vi "Set Exclusions By Path.vi"(8 "error in (no error)":errorcluster, 10 "Path exclusions":T1={"Exclude files from vi.lib"=TRUE, "Exclude files from instr.lib"=TRUE, "Exclude files from user.lib"=TRUE}, 11 "SDIST in":refnum<class "NI_AB_API_DSDIST.lvclass">) -> (0 "error out":errorcluster, 3 "SDIST out":refnum<class "NI_AB_API_DSDIST.lvclass">)   [LabVIEW 2020, in "NI_AB_API_DSDIST.lvclass"]
uses:
  <vilib>/AppBuilder/AB_API/DSDIST/NI_AB_API_DSDIST.lvclass
  <vilib>/AppBuilder/AB_API/common/AB_API Path Exclusions.ctl
  <vilib>/AppBuilder/AB_API/SDIST/NI_AB_API_SDIST.lvclass
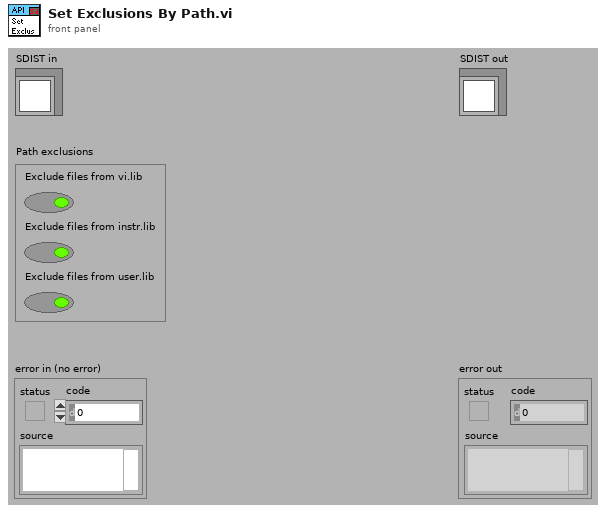
[diagram p1: front panel]
types:
  T1 = typedef "AB_API Path Exclusions.ctl" = cluster{"Exclude files from vi.lib":bool, "Exclude files from instr.lib":bool, "Exclude files from user.lib":bool}
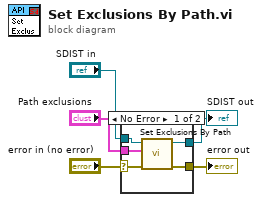
[diagram p0: block diagram]
diagram:
  n1 = case shown="No Error" "error in (no error)" {
    selector: "error in (no error)" -> [w10 w12]
    tunnel: [w9 w12] -> w4
    tunnel: [w7 w11] -> w2
    tunnel: "SDIST in" -> [w6 w11]
    tunnel: "Path exclusions" -> [w8 _]
    frame No Error {
      n2 = call-parent "Set Exclusions By Path.vi"("error in (no error)"=w10, "Path exclusions"=w8, "SDIST in"=w6) -> ("error out"=w9:errorcluster, "SDIST out"=w7:refnum<class "NI_AB_API_DSDIST.lvclass">)  [unwired: 7 in]
    }
    frame Error {
    }
  }
  "error out" <- w4
  "SDIST out" <- w2
